vi "Write Mode.vi"(8 "error in":errorcluster, 10 "Mode":T1, 11 "4081 in":refnum<class "4081.lvclass">) -> (0 "error out":errorcluster, 3 "4081 out":refnum<class "4081.lvclass">)   [LabVIEW 2019, in "4081.lvlib" / "4081.lvclass"]
uses:
  Library/4081.lvclass
  C:/Users/Public/Documents/Development/builds/Instruments/Multimeter.lvlibp/Library/Multimeter.lvclass
  builds/Instruments/Multimeter.lvlibp/Custom Controls/Mode.ctl
  Library/4081.lvclass/4081.ctl
  Read Local Resource.vi
  Write Local Resource.vi
  builds/Instruments/Multimeter.lvlibp/Accessors/Read Range.vi
  <instrlib>/niDMM/nidmm.llb/niDMM Configure Measurement Digits.vi
  builds/Instruments/Multimeter.lvlibp/Library/Multimeter.lvclass
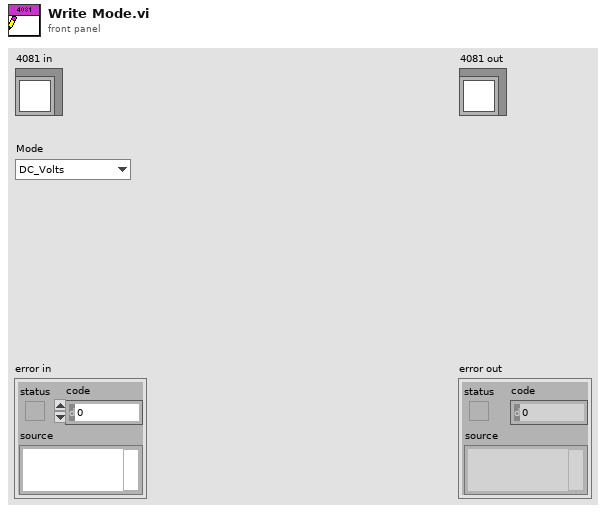
[diagram p1: front panel]
types:
  T1 = typedef "Multimeter.lvlibp/Multimeter.lvclass/Mode.ctl" = enum16{"DC_Volts", "AC_Volts", "DC_Current", "AC_Current", "Resistance_2_Wire", "Resistance_4_Wire", "Diode", "Frequency", "Period", "AC_Volts_DC_Coupled", "Capacitance", "Inductance", "Temperature"}
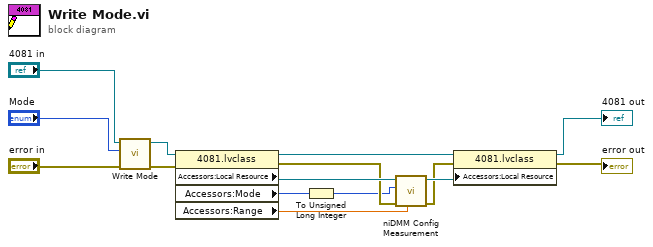
[diagram p0: block diagram]
diagram:
  n1 = call-parent "Write Mode.vi"("error in (no error)"="error in", "Mode"="Mode", "Multimeter in"="4081 in") -> ("error out"=w12:errorcluster, "Multimeter out"=w11:refnum<class "4081.lvclass">)  [unwired: 7 in]
  n2 = property class="4081.lvclass"(reference=w11, error in=w12) -> (reference out=w8:refnum<class "4081.lvclass">, error out=w4:errorcluster, "Accessors:Local Resource"=w10:refnum<k15>, "Accessors:Mode"=w7:T1, "Accessors:Range"=w1:dbl)
  n3 = To Unsigned Long Integer(number=w7) -> (unsigned 32bit integer=w2:u32)
  n4 = call-poly <instrlib>:"niDMM Config Measurement.vi"("Range"=w1, "error in (no error)"=w4, "Function"=w2, "instrument handle"=w10) -> ("error out"=w3:errorcluster, "instrument handle out"=w9:refnum<k15>)  [unwired: 6 in]
  n5 = property class="4081.lvclass"(reference=w8, error in=w3, "Accessors:Local Resource"=w9) -> (reference out=→"4081 out":refnum<class "4081.lvclass">, error out=→"error out":errorcluster)
